vi "niHWS Set Wfm DBL Attribute.vi"(8 "error in (no error)":errorcluster, 9 "attribute value":dbl format="%0.2f", 10 "attribute ID":T1 items=["X Axis Start"=0, "X Axis Increment"=1, "Y Axis Minimum"=3, "Y Axis Maximum"=4], 11 "waveform reference in":u32) -> (0 "error out":errorcluster, 3 "waveform reference out":u32)   [LabVIEW 2013]
doc: "Sets floating point attributes that apply to the waveform specified by the waveform reference."
uses:
  niHWS Set Wfm DBL Attribute ID.ctl
  nihwsu.dll
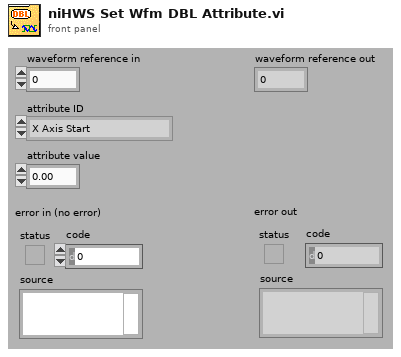
[diagram p1: front panel]
types:
  T1 = typedef "niHWS Set Wfm DBL Attribute ID.ctl" = u32
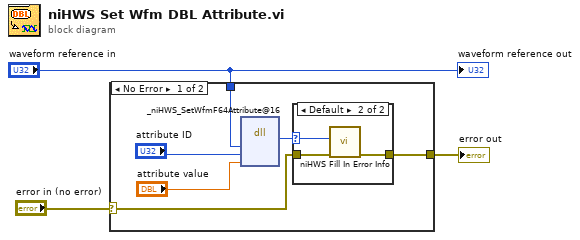
[diagram p0: block diagram]
diagram:
  n1 = case shown="No Error" "error in (no error)" {
    selector: "error in (no error)" -> [w5 w14]
    tunnel: [w6 w14] -> w3
    tunnel: "waveform reference in" -> [w7 _]
    frame No Error {
      n2 = dll-call lib="nihwsu.dll" fn="_niHWS_SetWfmF64Attribute@16"("wfmReference"=w7, "attributeID"="attribute ID", "attributeVal"="attribute value") -> (w4:i32)  [unwired: 6 in, 2 out]
      n3 = case shown="Default" w4 {
        selector: w4 -> [_ w11]
        tunnel: [w10 w12] -> w6
        tunnel: w5 -> [w10 w13]
        frame 0 {
        }
        frame Default {
          n4 = call "niHWS Fill In Error Info.vi"("error in (no error)"=w13, "status code"=w11) -> ("error out"=w12:errorcluster)  [unwired: 9 in]
        }
      }
    }
    frame Error {
    }
  }
  "error out" <- w3
  "waveform reference out" <- "waveform reference in"
